vi "view debug.vi"() -> ()   [LabVIEW 2022 SP3]
uses:
  View/Serial port assistant view.lvclass
panel:
  out "Request":string
  out "Model Number":i32
  out "Model Name":string
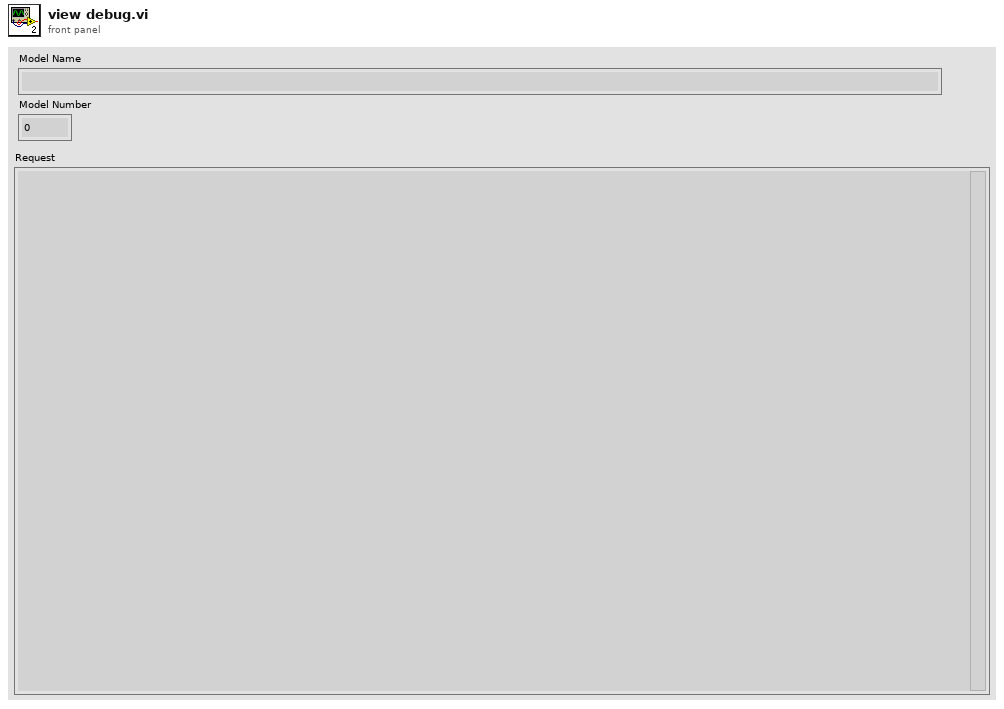
[diagram p1: front panel]
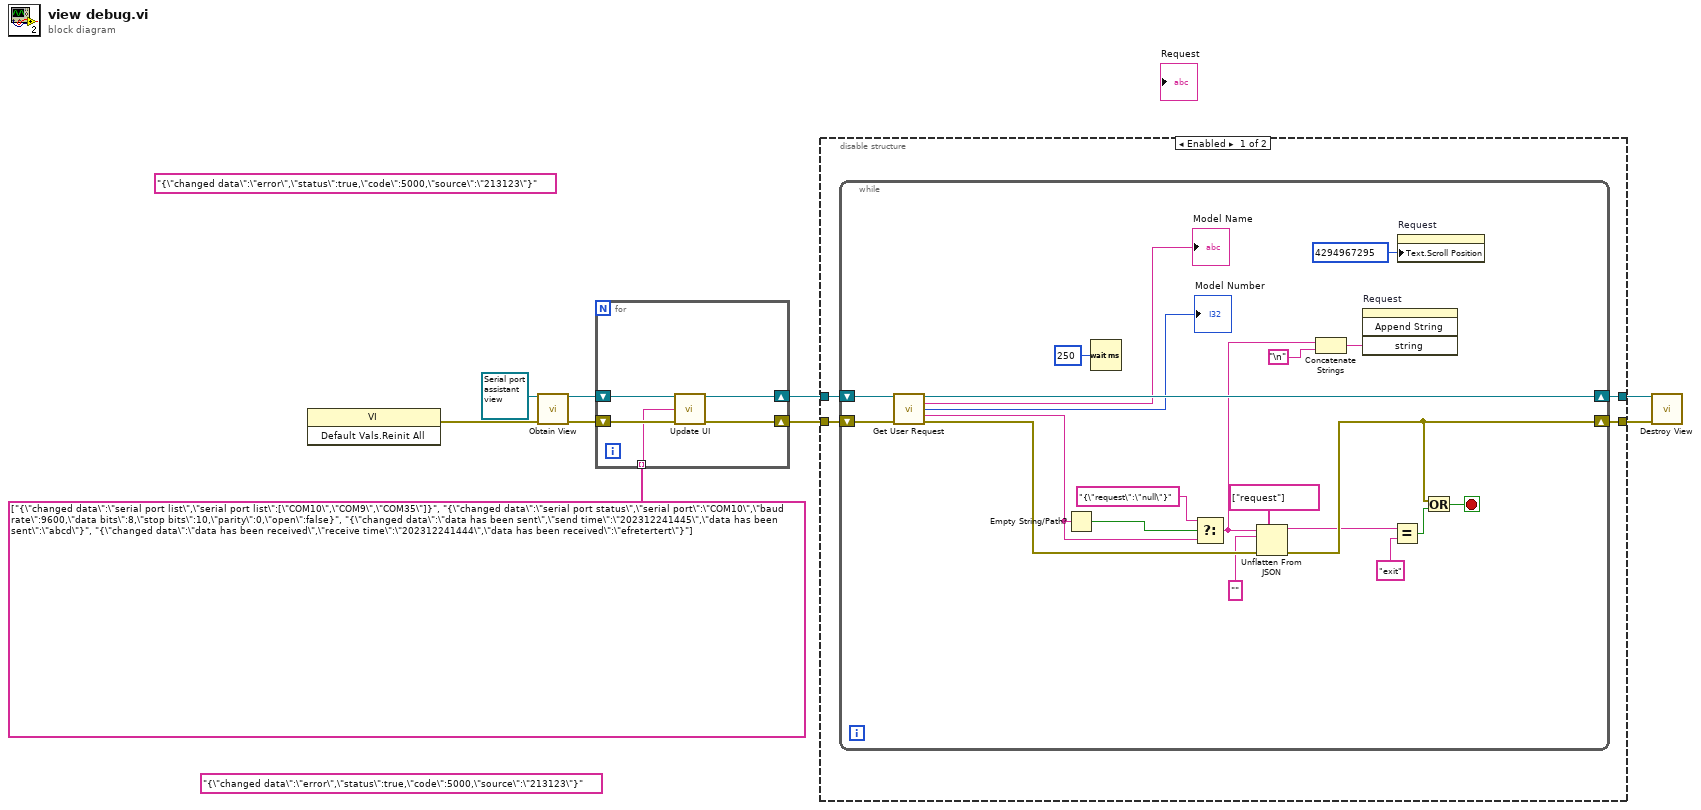
[diagram p0: block diagram]
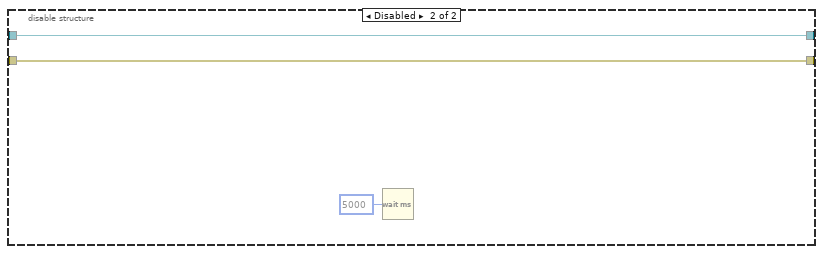
[diagram p2: hidden frame]
diagram:
  (unwired) "{\"changed data\":\"error\",\"status\":true,\"code\":5000,\"source\":\"213123\"}"
  (unwired) "{\"changed data\":\"error\",\"status\":true,\"code\":5000,\"source\":\"213123\"}"
  n1 = invoke class="VI" method="Default Vals.Reinit All"() -> (error out=w1:errorcluster)  [unwired: 3 in, 2 out]
  n2 = call-dynamic "Obtain View.vi"("Serial port assistant view in"=refnum<class "Serial port assistant view.lvclass"> refnum, "error in (no error)"=w1) -> ("Serial port assistant view out"=w5:refnum<class "Serial port assistant view.lvclass">, "error out"=w6:errorcluster)  [unwired: 12 in]
  n3 = for {
    shift-right: [w12] -> w4
    shift-left: w5 -> [w14]
    shift-right: [w11] -> w3
    shift-left: w6 -> [w13]
    tunnel: string[] ["{\"changed data\":\"serial port list\",\"serial port list\":[\"COM10\",\"COM9\",\"COM35\"]}", "{\"changed data\":\"serial port status\",\"serial port\":\"COM10\",\"baud rate\":9600,\"data bits\":8,\"stop bits\":10,\"parity\":0,\"open\":false}", "{\"changed data\":\"data has been sent\",\"send time\":\"202312241445\",\"data has been sent\":\"abcd\"}", "{\"changed data\":\"data has been received\",\"receive time\":\"202312241444\",\"data has been received\":\"efretertert\"}"] -> [w10] mode=indexing
    n4 = call-dynamic "Update UI.vi"("Serial port assistant view in"=w14, "changed data"=w10, "error in (no error)"=w13) -> ("Serial port assistant view out"=w12:refnum<class "Serial port assistant view.lvclass">, "error out"=w11:errorcluster)  [unwired: 11 in]
  }
  n5 = disable-structure shown="Enabled" {
    disable-tunnel: [w18 w41] -> w8
    disable-tunnel: [w17 w42] -> w7
    disable-tunnel: w4 -> [w16 w42]
    disable-tunnel: w3 -> [w15 w41]
    frame Enabled {
      n6 = while {
        shift-right: [w39] -> w17
        shift-left: w16 -> [w20]
        shift-right: [w24] -> w18
        shift-left: w15 -> [w19]
        stop <- w34 stop-if-true
        n7 = call-dynamic "Get User Request.vi"("Serial port assistant view in"=w20, "error in (no error)"=w19) -> ("Serial port assistant view out"=w39:refnum<class "Serial port assistant view.lvclass">, "Model Name"=→"Model Name":string, "Model Number"=→"Model Number":i32, "Request"=w25:string, "error out"=w36:errorcluster)  [unwired: 9 in]
        n8 = Empty String/Path?(string/path=w25) -> (empty?=w28:bool)
        n9 = Wait (ms)(milliseconds to wait=u32 250) -> ()  [unwired: 1 out]
        n10 = Select(t="{\"request\":\"null\"}", s=w28, f=w25) -> (s? t:f=w21:string)
        n11 = Unflatten From JSON(path=string[] ["request"], JSON string=w21, type and defaults="", error in (no error)=w36) -> (value=w23:string, error out=w24:errorcluster)  [unwired: 3 in]
        n12 = Concatenate Strings(w21, "\n") -> (w30:string)
        n13 = invoke on="Request" class="Str" method="Append String"("string"=w30) -> ()  [unwired: 3 in, 4 out]
        n14 = Equal?(x=w23, y="exit") -> (x = y?=w35:bool)
        n15 = property on="Request" class="Str"("Text.Scroll Position"=u32 4294967295) -> ()  [unwired: 2 in, 2 out]
        n16 = Or(x=w24, y=w35) -> (x .or. y?=w34:bool)
      }
    }
    frame Disabled {
      n17 = Wait (ms)(milliseconds to wait=u32 5000) -> ()  [unwired: 1 out]
    }
  }
  n18 = call-dynamic "Destroy View.vi"("Serial port assistant view in"=w7, "error in (no error)"=w8) -> ()  [unwired: 12 in, 2 out]
